vi "Sub Initialize.vi"(6 "Controller name":string, 8 "error in (no error)":errorcluster, 11 "Stepper in":refnum<class "Stepper.lvclass">) -> (0 "error out":errorcluster, 2 "Initialize Result":refnum<class "Acquired Result.lvclass">, 3 "Stepper out":refnum<class "Stepper.lvclass">)   [LabVIEW 2021, in "Stepper.lvclass"]
uses:
  Stepper.lvclass
  C:/Program Files/National Instruments/LabVIEW 2021/vi.lib/ActorFramework/Actor/Actor.lvclass
  NHMFL_Core/Libraries/Instruments/Results/Acquired Result/Acquired Result.lvclass
  <vilib>/ActorFramework/Actor/Actor.lvclass/Actor.ctl
  <vilib>/ActorFramework/Message Enqueuer/Message Enqueuer.lvclass/Message Enqueuer.ctl
  <vilib>/ActorFramework/Message Enqueuer/Init from Existing Queue.vi
  Measurements/Response Synchronizer/Response Synchronizer.lvclass
  <vilib>/ActorFramework/Message Enqueuer/Message Enqueuer.lvclass
  Continuous Recorder Actor/Continuous Recorder Actor.lvclass
  Stepper.lvclass/Stepper.ctl
  <vilib>/ActorFramework/Actor/Actor.lvclass
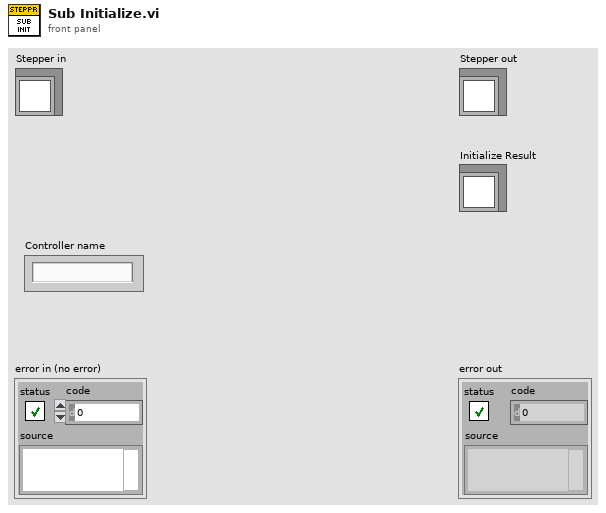
[diagram p1: front panel]
types:
  T1 = typedef "Stepper Config.ctl" = cluster{"Start":dbl, "End":dbl, "Step":dbl, "Append measurements":string[]}
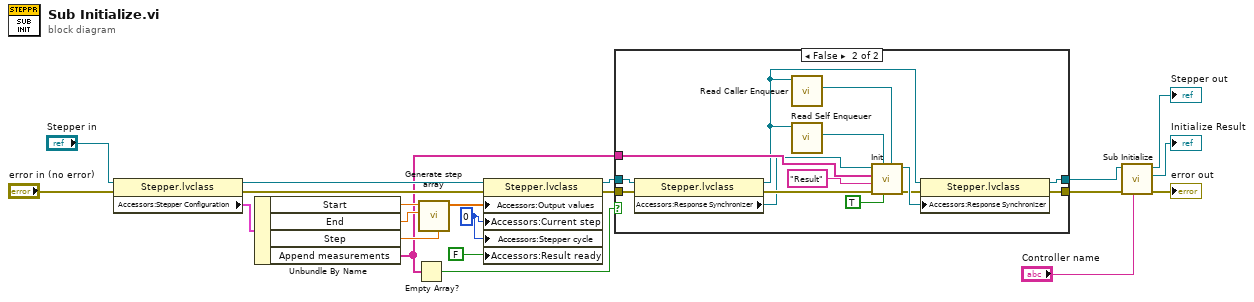
[diagram p0: block diagram]
diagram:
  w1 = 0 ("Current step")
  n1 = property class="Stepper.lvclass"(reference="Stepper in", error in="error in (no error)") -> (reference out=w8:refnum<class "Stepper.lvclass">, error out=w9:errorcluster, "Accessors:Stepper Configuration"=w10:T1)
  n2 = Unbundle By Name(w10) -> ("Start"=w16:dbl, "End"=w15:dbl, "Step"=w14:dbl, "Append measurements"=w3:string[])
  n3 = Empty Array?(array=w3) -> (empty?=w17:bool)
  n4 = call "Generate step array.vi"("Step"=w14, "End"=w15, "Start"=w16) -> ("Steps"=w11:dbl[])  [unwired: 8 in]
  n5 = property class="Stepper.lvclass"(reference=w8, error in=w9, "Accessors:Output values"=w11, "Accessors:Current step"=w1, "Accessors:Stepper cycle"=w1, "Accessors:Result ready"=FALSE ("Result ready")) -> (reference out=w12:refnum<class "Stepper.lvclass">, error out=w13:errorcluster)
  n6 = case shown="False" w17 {
    tunnel: [w23 w26] -> w7
    tunnel: w13 -> [w22 w32]
    tunnel: [w22 w24] -> w4
    tunnel: w3 -> [_ w35]
    tunnel: w12 -> [w23 w30]
    frame True {
    }
    frame False {
      n7 = property class="Stepper.lvclass"(reference=w30, error in=w32) -> (reference out=w27:refnum<class "Stepper.lvclass">, error out=w31:errorcluster, "Accessors:Response Synchronizer"=w29:refnum<class "Response Synchronizer.lvclass">)
      n8 = call <vilib>:"Read Caller Enqueuer.vi"("Actor"=w27) -> ("Caller Enqueuer"=w34:refnum<class "Message Enqueuer.lvclass">)  [unwired: 10 in]
      n9 = call <vilib>:"Read Self Enqueuer.vi"("Actor"=w27) -> ("Self Enqueuer"=w33:refnum<class "Message Enqueuer.lvclass">)  [unwired: 10 in]
      n10 = call-dynamic "Init.vi"("Caller Enqueuer"=w34, "Subscribe"=TRUE, "Self Enqueuer"=w33, "error in (no error)"=w31, "Topic"="Result", "Responder names"=w35, "Response Synchronizer in"=w29) -> ("error out"=w25:errorcluster, "Response Synchronizer out"=w28:refnum<class "Response Synchronizer.lvclass">)  [unwired: 3 in]
      n11 = property class="Stepper.lvclass"(reference=w27, error in=w25, "Accessors:Response Synchronizer"=w28) -> (reference out=w26:refnum<class "Stepper.lvclass">, error out=w24:errorcluster)
    }
  }
  n12 = call-parent "Sub Initialize.vi"("Controller name"="Controller name", "error in (no error)"=w4, "Instrument Recorder in"=w7) -> ("error out"=→"error out":errorcluster, "Initialize Result"=→"Initialize Result":refnum<class "Acquired Result.lvclass">, "Instrument Recorder out"=→"Stepper out":refnum<class "Stepper.lvclass">)  [unwired: 6 in]
